vi "InitializeTDMS.vi"(7 "FilePath":path, 8 "error in (no error)":errorcluster, 9 "Images per File":i64, 11 "Image Ref in":T3) -> (0 "error out":errorcluster, 1 "Write Settings Out":T2 {"Image Type" items=["Grayscale (U8)", "Grayscale (I16)", "Grayscale (SGL)", "Complex (CSG)", "RGB (U32)", "HSL (U32)", "RGB (U64)", "Grayscale (U16)"]}, 2 "Optimizations":T4, 3 "Refnum out":refnum<k34>)   [LabVIEW 2024]
uses:
  <vilib>/vision/Image Controls.llb/IMAQ Image.ctl
  TDMS Write Settings.ctl
  TDMS File Initialization (Write).vi
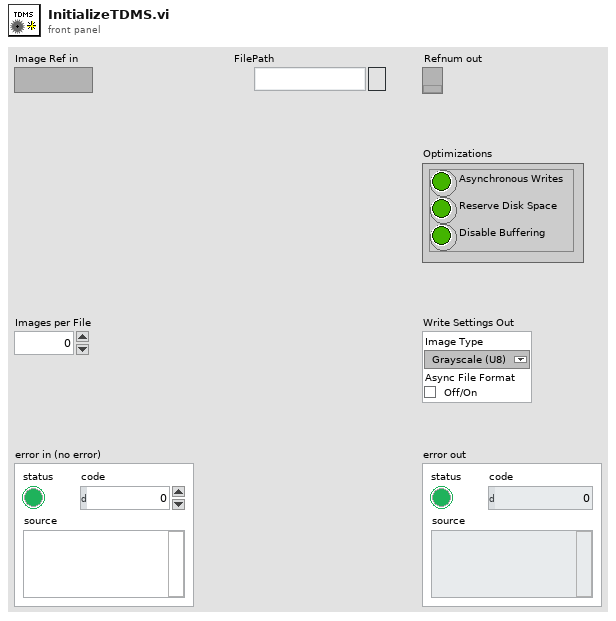
[diagram p1: front panel]
types:
  T1 = typedef "Image Type" = u32
  T2 = cluster{"Image Type":T1, "Async File Format":bool}
  T3 = typedef "IMAQ Image.ctl" = refnum<image>
  T4 = cluster{"Asynchronous Writes":bool, "Reserve Disk Space":bool, "Disable Buffering":bool}
  T5 = typedef "TDMS Write Settings.ctl" = cluster{"Asynchronous":bool, "Disable Buffering if Supported":bool, "Reserved Images":i64, "Fail if Reservation Fails":bool}
  T6 = cluster{"Asynchronous Write":bool, "Reserve Disk Space":bool, "Disable Buffering":bool}
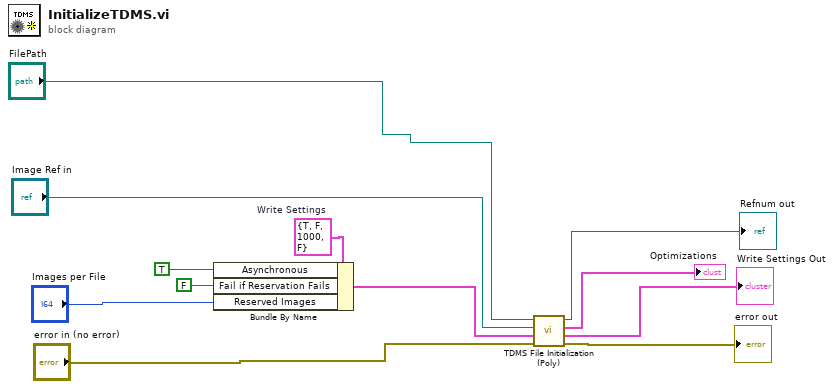
[diagram p0: block diagram]
diagram:
  w8 = T5 {"Asynchronous"=TRUE, "Disable Buffering if Supported"=FALSE, "Reserved Images"=1000, "Fail if Reservation Fails"=FALSE}  # Write Settings
  n1 = Bundle By Name(cluster=w8, "Asynchronous"=TRUE, "Fail if Reservation Fails"=FALSE, "Reserved Images"="Images per File") -> (w6:T5)
  n2 = call-poly "TDMS File Initialization (Poly).vi"("error in (no error)"="error in (no error)", "Write Settings"=w6, "Image In"="Image Ref in", "File Path"="FilePath") -> ("error out"=→"error out":errorcluster, "Write Settings Out"=→"Write Settings Out":T2, "Optimizations Configured"=→"Optimizations":T6, "TDMS Refnum Out"=→"Refnum out":refnum<k34>)  [unwired: 4 in]
